vi "checkCalistatus.vi"(8 "error in":errorcluster, 10 "DBSet":T1, 11 "SystemMode":string) -> (1 "calibrated?":bool)   [LabVIEW 2011]
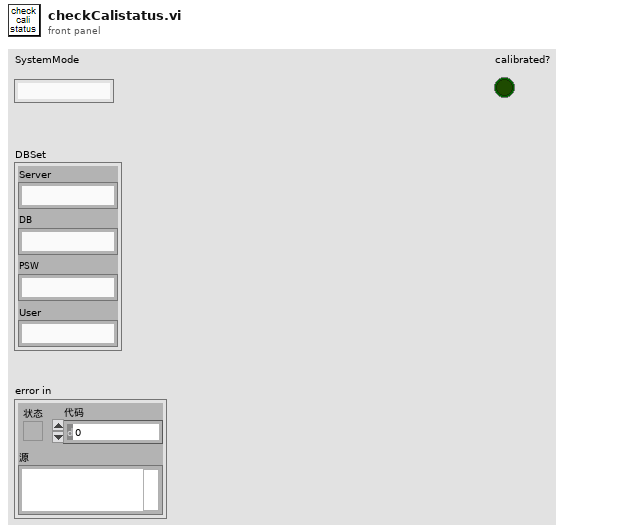
[diagram p1: front panel]
types:
  T1 = cluster{"Server":string, "DB":string, "PSW":string, "User":string}
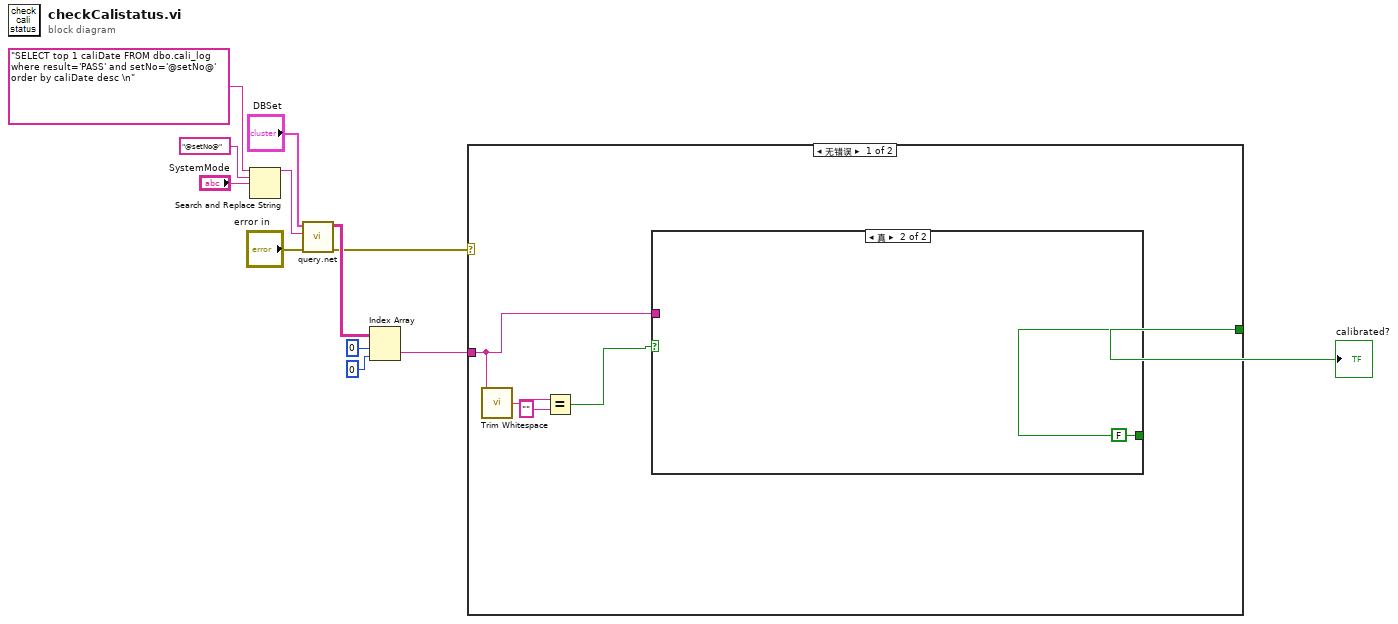
[diagram p0: block diagram]
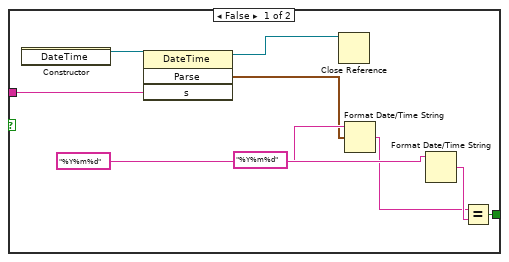
[diagram p2: hidden frame]
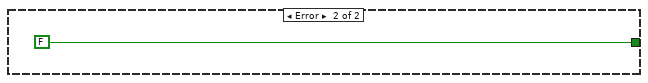
[diagram p3: hidden frame]
diagram:
  n1 = Search and Replace String(input string="SELECT top 1 caliDate FROM dbo.cali_log where result='PASS' and setNo='@setNo@' order by caliDate desc \n", search string="@setNo@" ("搜索字符串"), replace string="SystemMode") -> (result string=w9:string)  [unwired: 5 in, 3 out]
  n2 = call "query.net.vi"("错误输入（无错误）"="error in", "Sql"=w9, "DBSet"="DBSet") -> ("错误输出"=w2:errorcluster, "result"=w7:string[][])  [unwired: 7 in]
  n3 = Index Array(array=w7, index (row)=0 ("索引 (行)"), index (col)=0 ("禁用的索引 (列)")) -> (element=w1:string)
  n4 = case shown="无错误" w2 {
    tunnel: [w17 FALSE] -> w4
    tunnel: w1 -> [w16 _]
    frame No Error {
      n5 = call <vilib>:"Trim Whitespace.vi"("string"=w16) -> ("trimmed string"=w15:string)  [unwired: 1 in]
      n6 = Equal?(x=w15, y="") -> (x = y?=w13:bool)
      n7 = case shown="真" w13 {
        tunnel: [w24 FALSE] -> w17
        tunnel: w16 -> [w18 _]
        frame False {
          n8 = constructor class="DateTime"() -> (reference out=w20:refnum<k24>)  [unwired: 3 in, 2 out]
          n9 = invoke class="DateTime" method="Parse"(reference=w20, "s"=w18) -> (reference out=w23:refnum<k24>, "Parse"=w21:timestamp)  [unwired: 2 in, 2 out]
          n10 = Close Reference(reference=w23) -> ()  [unwired: 1 in, 1 out]
          n11 = Format Date/Time String(time format string (%c)="%Y%m%d" ("时间格式字符串(%c)"), seconds (now)=w21) -> (date/time string=w19:string)  [unwired: 1 in]
          n12 = Format Date/Time String(time format string (%c)="%Y%m%d" ("时间格式字符串(%c)")) -> (date/time string=w25:string)  [unwired: 2 in]
          n13 = Equal?(x=w19, y=w25) -> (x = y?=w24:bool)
        }
        frame True {
        }
      }
    }
    frame Error {
    }
  }
  "calibrated?" <- w4
